vi "Mutation v3.vi"(9 "Mutation probability":dbl=0.01 min=0.0 max=1.0 step=0.1, 11 "Path In":T1={"Distance"=0.0, "Tour"=[1, 14, 13, 12, 7, 6, 15, 5, 11, 9, 10, 16, 3, 2, 4, 8, 1]}) -> (3 "Path Out":T1={"Distance"=0.0, "Tour"=[68, 82, 14, 66, 38, 76, 91, 89, 87, 84, 25, 25, 88]})   [LabVIEW 2015, in "TSP Library.lvlib"]
uses:
  TSP Library.lvlib
  TypeDef/Path.ctl
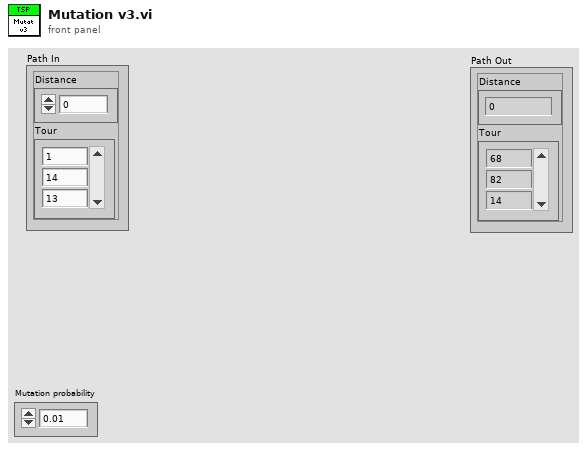
[diagram p1: front panel]
types:
  T1 = typedef "TSP Library.lvlib/Path.ctl" = cluster{"Distance":dbl, "Tour":u16[]}
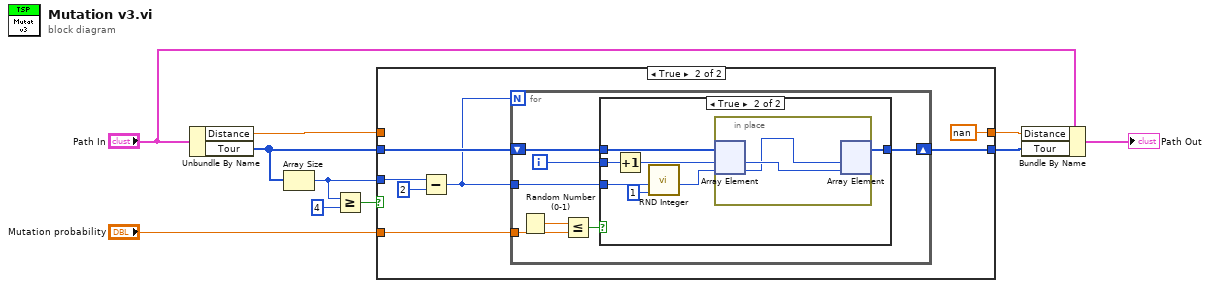
[diagram p0: block diagram]
diagram:
  n1 = Unbundle By Name("Path In") -> ("Distance"=w3:dbl, "Tour"=w1:u16[])
  n2 = Array Size(array=w1) -> (size(s)=w6:i32)
  n3 = Greater Or Equal?(x=w6, y=4) -> (x >= y?=w4:bool)
  n4 = case shown="True" w4 {
    tunnel: [w12 w16] -> w8
    tunnel: w1 -> [w12 w19]
    tunnel: "Mutation probability" -> [_ w14]
    tunnel: w6 -> [_ w17]
    tunnel: w3 -> [w11 _]
    tunnel: [w11 nan ("Distance")] -> w2
    frame False {
    }
    frame True {
      n5 = Subtract(x=w17, y=2) -> (x-y=w13:i32)
      n6 = for {
        N: w13 -> [_]
        shift-right: [w25] -> w16
        shift-left: w19 -> [w26]
        tunnel: w13 -> [w20]
        tunnel: w14 -> [w23]
        i -> [w21]
        n7 = Random Number (0-1)() -> (number: 0 to 1=w24:dbl)
        n8 = Less Or Equal?(x=w24, y=w23) -> (x <= y?=w22:bool)
        n9 = case shown="True" w22 {
          tunnel: w26 -> [w27 w34]
          tunnel: [w27 w33] -> w25
          tunnel: w21 -> [_ w32]
          tunnel: w20 -> [_ w30]
          frame False {
          }
          frame True {
            n10 = Increment(x=w32) -> (x+1=w31:i32)
            n11 = call "RND Integer.vi"("Min"=1, "Max"=w30) -> ("RND Integer"=w28:i32)  [unwired: 9 in]
            n12 = in-place {
              n13 = in-place-array #1(w34, w31, w28) -> (w36:u16, w35:u16)
              n14 = in-place-array #1(w35, w36) -> (w33:u16[])  [unwired: 2 out]
            }
          }
        }
      }
    }
  }
  n15 = Bundle By Name(cluster="Path In", "Distance"=w2, "Tour"=w8) -> (→"Path Out":T1)
